vi "Strain Gauge Motion [FPGA Main].vi"() -> ()   [LabVIEW 2017]
doc: "Use this VI to control the cRIO Demo Kit motor and motor drive with a simple set of commands. You can operate the drive in 2 different modes. By default, you can input a velocity setpoint withing +20 or -20 rotations per second and the motor will move to that velocity, limited by the maximum acceleration input. Alternatively, you can turn on the heater mode. This will use the motor like a heater coil within the demo kit by setting the velocity to zero, but enabling full holding current through the drive. You can use the thermocouple in the demo kit to read the temperature of the motor windings. Turn the heating coil on and off by enabling and disabling the drive.\n\nUSING THIS VI: You can run this VI as the top level VI for an easy motion or heater component. Or you can modify this VI to run as a component of a main FPGA application. To do this, replace the front panel objects with target scoped registers, UDVs, or global variables."
uses:
  <vilib>/Platform/TimedLoop/XDataNode/timing_clust.ctl
  <vilib>/Platform/TimedLoop/XDataNode/nitl_modes.ctl
  <vilib>/Platform/TimedLoop/XDataNode/wakeup.ctl
  <vilib>/Motion/MotorControl/_s/nism.encoder.incremental.config.ctl
  <vilib>/Motion/MotorControl/_s/nism.incremental.indexCriteria.ctl
  <vilib>/LabVIEW Targets/FPGA/cRIO/shared/nicrio_ModuleControls/nicrio_cRIO-9503_DriveStatus.ctl
  <vilib>/Motion/MotorControl/_s/nism.stepper.currentScheduler.config.ctl
  <vilib>/Motion/MotorControl/_s/nism.microstepping.rate.ctl
  <vilib>/Motion/MotorControl/_s/nism.pi.gains.sgl.ctl
  <vilib>/Motion/MotorControl/_s/nism.pi.c.currentFeedback.sgl.ctl
  <vilib>/Motion/MotorControl/_s/nism.mdo.antiResonanceData.ctl
  <vilib>/Motion/MotorControl/_s/nism.stepper.currentScheduler.torqueSmoothingCoefficients.ctl
  <vilib>/Motion/MotorControl/_s/nism.pwm.outputs.4phase.ctl
  <vilib>/rvi/Emulation/niFpgaGetClockAttributes.vi
  <vilib>/rvi/Emulation/niFpgaSctlEmulationGetInTimedLoop.vi
  <vilib>/rvi/Emulation/niFpgaEmulationReportErrorSimple.vi
  <vilib>/rvi/eio/common/nirviEmuTemplateMethod_errors.vi
  <vilib>/rvi/Emulation/niFpgaCriticalErrorInLSC.vi
  <vilib>/rvi/DataTransferAndStorage/Container/Common/niFpgaContainerGetUniqueNameForEmu.vi
  <vilib>/rvi/DataTransferAndStorage/Container/Common/niFpgaContainerSetEmuInfo.vi
  <vilib>/rvi/eio/common/nirviEmuReportErrorAndStop.vi
  <vilib>/rvi/Emulation/niFpgaProcessEmulError.vi
  <vilib>/rvi/Emulation/niFpgaEmulationIsFPGAContextNoSignature.vi
  <vilib>/rvi/Memory/Memory_Emulation/niFpgaMemoryEmulationCacheClearOnFirstRun.vi
  <vilib>/rvi/Memory/Memory_Emulation/nirvimemoryEmulationManagerCache_MakeExclusive.vi
  <vilib>/rvi/Memory/Memory_Emulation/niFpgaMemoryEmulationValidateCache.vi
  <vilib>/rvi/Memory/Memory_Emulation/nirvimemoryEmulationManagerCache_InsertValue.vi
  <vilib>/Utility/error.llb/Clear Errors.vi
  <vilib>/rvi/Memory/Memory_Emulation/nirvimemoryEmulationManagerCache_ReleaseExclusive.vi
  <vilib>/rvi/Memory/Memory_Emulation/nirvimemoryEmulationManagerCache_GetValue.vi
  <vilib>/rvi/Memory/Memory_Emulation/nirvimemoryEmulationManagerCache_SetValue.vi
  <vilib>/Motion/MotorControl/_s/nism.incremental.p.2.vi
  <vilib>/rvi/occurrence/nirviWaitOnOccurrenceBase.vi
  <vilib>/Motion/MotorControl/_s/nism.rateLimiter.v.fxp.vi
  <vilib>/Motion/MotorControl/_s/nism.stepResolver.fxp.64.32.vi
  <vilib>/Motion/MotorControl/_s/nism.stepper.currentScheduler.advanced.single.vi
  <vilib>/Motion/MotorControl/_s/nism.pi.c.sgl.2phase.2.noAW.vi
  <vilib>/Motion/MotorControl/_s/nism.antiResonance.single.vi
  <vilib>/Motion/MotorControl/_s/nism.9503VoltageTransform.fxp.vi
  <vilib>/eio/EIONode/EIONode.xnode
  <vilib>/rvi/LocalResourceManager/LocalResourceManager.xnode
  <vilib>/rvi/DataTransferAndStorage/Container/XNode/niFpgaContainer.xnode
  <vilib>/rvi/DataTransferAndStorage/Register/Emulation/niFpgaRegisterEmulation.vi
  <vilib>/eio/EIOMethodNode/EIOMethodNode.xnode
  <vilib>/platform/TimedLoop/XDataNode/XDataNode.xnode
  <vilib>/Motion/MotorControl/NI_SoftMotion_MotorControlIP.lvlib
  <vilib>/Platform/TimedLoop/XDataNode/XDNodeRunTimeDep.lvlib
panel:
  out "Strain Gauge":sgl
  in  "Heater Mode":bool
  in  "Velocity Setpoint (rev/sec)":sgl caption="velocity setpoint"
  in  "Maximum Acceleration":T1(ring)=enum."High"
  out "Control Loop Timer":u32
  out "Anti-Resonance Enabled?":bool
  out "Pulse Per Revolution":bool
  out "Velocity (rev/sec)":fxp<+/-,32,16> caption="xi" format="%.41g"
  in  "Clear Faults":bool
  in  "Enable Drive":bool
  out "Module Fault Code":u16
  out "Module Fault?":bool
  # "Velocity is limited to +10 or -10 revolutions per second. Positive velocity setpoints equate to counter clockwise rotation.\n\nMax acceleration choices limit the rate of acceleration when changing velocity setpoints.\n\nHeater Mode will stop the motor and always keep full current through the motor windings, generating more heat.\n\nVelocity is the measured encoder velocity and works without the drive enabled. Pulse Per Revolution is the Z encoder pulse and occors exactly once for each revolution."
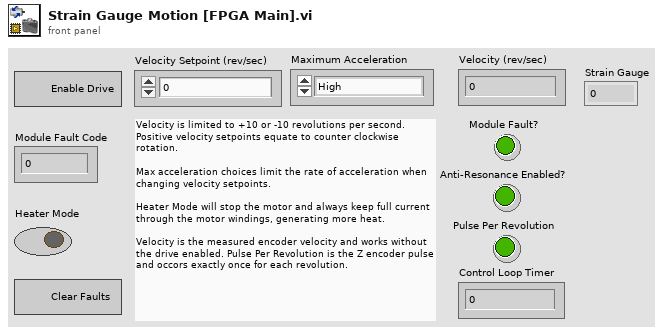
[diagram p1: front panel]
types:
  T1 = enum8{"Extremely Low", "Very Low", "Low", "Medium", "High", "Highest"}
  T2 = typedef "nicrio_cRIO-9503_DriveStatus.ctl" = enum8{"Drive Disabled (Disabled by fault)", "Drive Disabled (Disabled by software)", "Drive Enabled"}
  T3 = typedef "NI_SoftMotion_MotorControlIP.lvlib/nism.pwm.outputs.4phase.ctl" = cluster{"a+":fxp<+/-,16,1>, "a-":fxp<+/-,16,1>, "b+":fxp<+/-,16,1>, "b-":fxp<+/-,16,1>}
  T4 = typedef "XDNodeRunTimeDep.lvlib/timing_clust.ctl" = cluster{"Expected End [f-1]":u64, "Actual End [f-1]":u64, "Finished Late? [f-1]":bool, "Expected End [i-1]":u64, "Actual End [i-1]":u64, "Finished Late? [i-1]":bool, "Expected Start [i]":u64, "Actual Start [i]":u64, "Expected Start [f]":u64, "Actual Start [f]":u64, "Source Name":string, "Structure Name":string, "Period":i64, "Deadline":i64, "Offset":i64, "Start":i64, "Priority":i32, "Timeout":i32, "Mode":T5, "Wakeup Reason":T6, "Error":errorcluster, "Source Type":string, "Secondary Source Type":string, "Global End Time":u64, "Global Start Time":u64, "Frame Duration":u64, "Iteration Duration":u64, "Assigned CPU":i32, "I/O Scan Engine Mode":u32}
  T5 = typedef "XDNodeRunTimeDep.lvlib/nitl_modes.ctl" = enum32{"No Change", "Process missed periods, maintain original phase", "Discard missed periods, maintain original phase", "Process missed periods, ignore original phase", "Discard missed periods, ignore original phase"}
  T6 = typedef "XDNodeRunTimeDep.lvlib/wakeup.ctl" = enum32{"Normal", "Aborted", "Asynchronous wakeup", "Timing source error", "Timed loop error", "Timeout"}
  T7 = typedef "NI_SoftMotion_MotorControlIP.lvlib/nism.encoder.incremental.config.ctl" = cluster{"line a active high?":bool, "line b active high?":bool, "index active high?":bool}
  T8 = typedef "NI_SoftMotion_MotorControlIP.lvlib/nism.incremental.indexCriteria.ctl" = cluster{"a":bool, "b":bool, "z":bool}
  T9 = typedef "NI_SoftMotion_MotorControlIP.lvlib/nism.stepper.currentScheduler.torqueSmoothingCoefficients.ctl" = cluster{"current scheduler : torque smoothing : torque smoothing gain":sgl, "torque smoothing phase":fxp<+/-,16,1>}
  T10 = typedef "NI_SoftMotion_MotorControlIP.lvlib/nism.mdo.antiResonanceData.ctl" = cluster{"coefficient 0":sgl, "coefficient 1":sgl, "coefficient 2":sgl, "coefficient 3":sgl, "coefficient 4":sgl, "coefficient 5":sgl}
  T11 = typedef "NI_SoftMotion_MotorControlIP.lvlib/nism.pi.c.currentFeedback.sgl.ctl" = cluster{"phase a":sgl, "phase b":sgl}
  T12 = typedef "NI_SoftMotion_MotorControlIP.lvlib/nism.pi.gains.sgl.ctl" = cluster{"kp":sgl, "ki":sgl}
  T13 = typedef "NI_SoftMotion_MotorControlIP.lvlib/nism.microstepping.rate.ctl" = enum8{"1 (Full Step)", "2 (Half Step)", "4", "8", "16", "32", "64", "128", "256"}
  T14 = typedef "NI_SoftMotion_MotorControlIP.lvlib/nism.stepper.currentScheduler.config.ctl" = cluster{"rated phase current":sgl, "phase current offset(a)":sgl, "phase current offset(b)":sgl, "reduced current":sgl, "curr. reduction del.":u16}
  T15 = typedef "NI_SoftMotion_MotorControlIP.lvlib/nism.pi.c.currentSetpoint.sgl.ctl" = cluster{"phase a":sgl, "phase b":sgl}
  T16 = typedef "NI_SoftMotion_MotorControlIP.lvlib/nism.pi.c.voltage.sgl.ctl" = cluster{"phase a":sgl, "phase b":sgl}
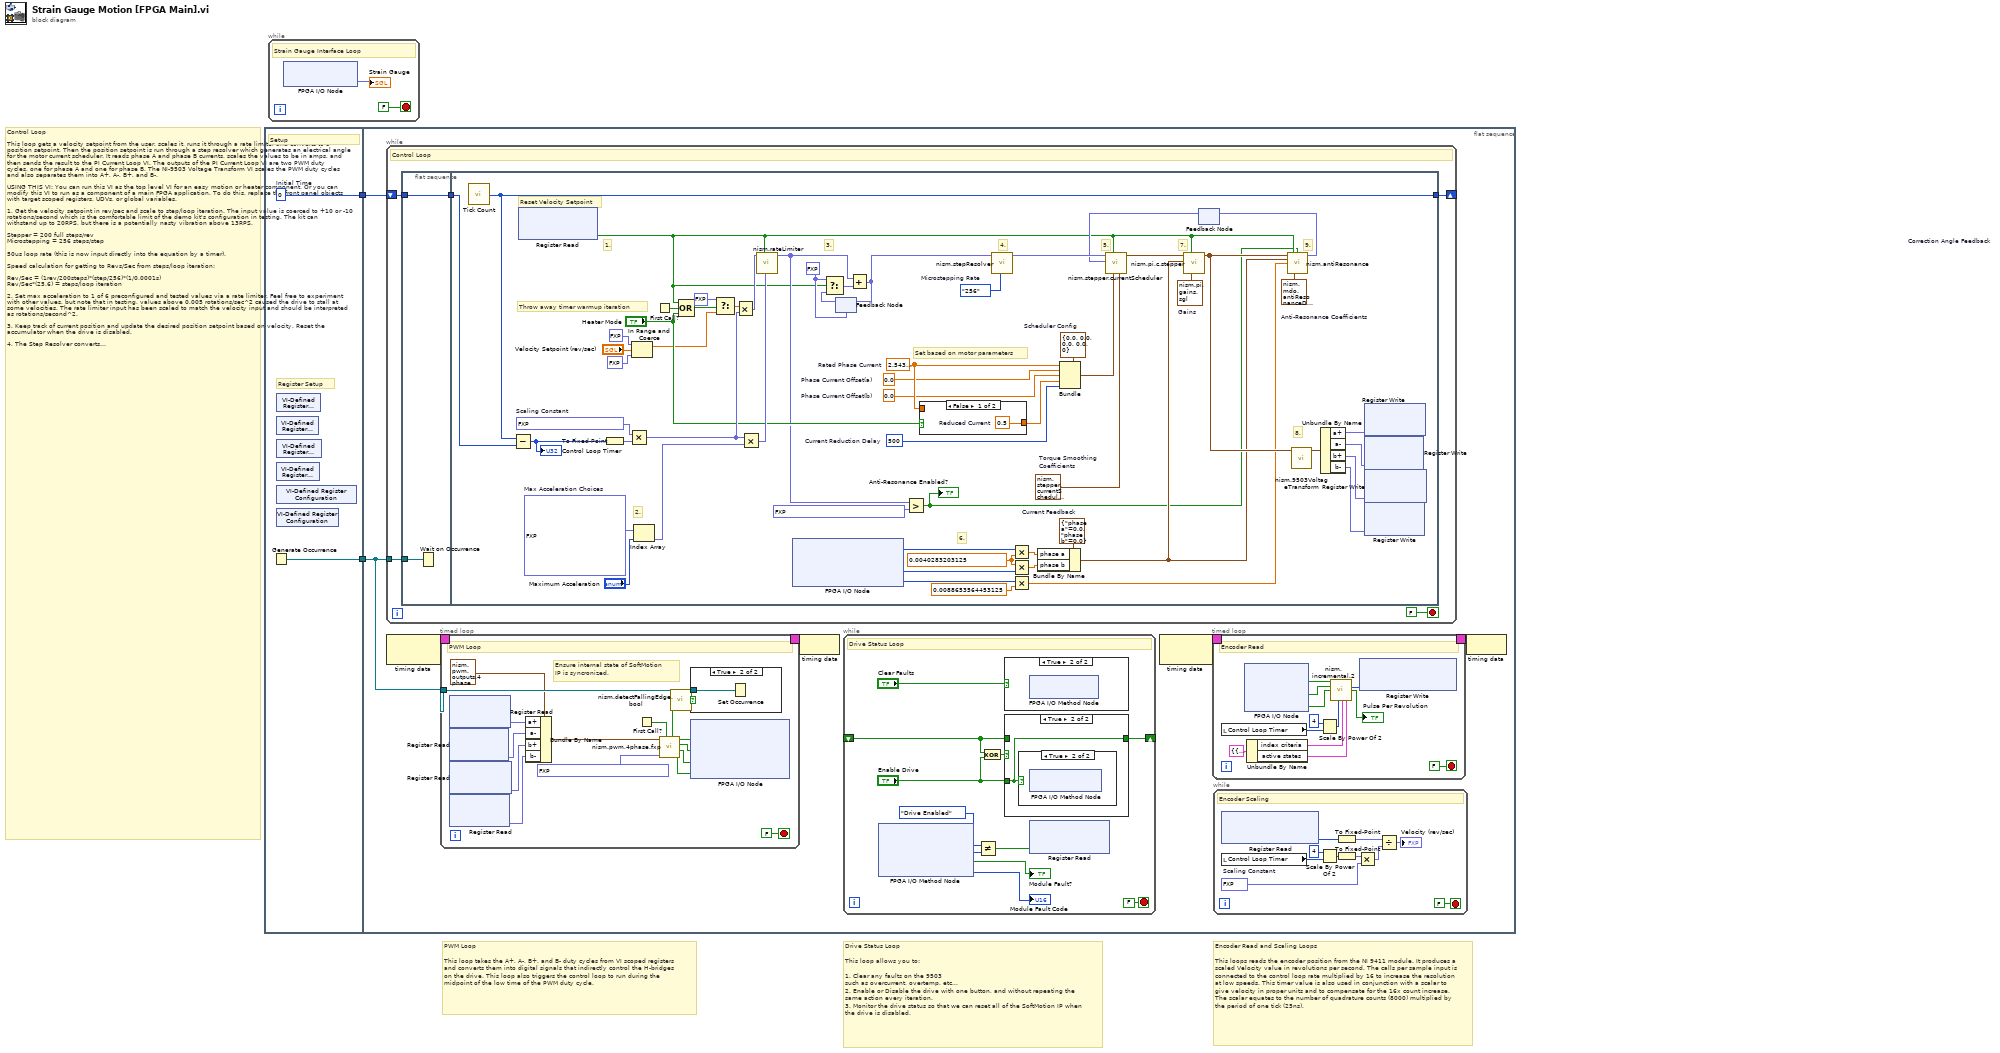
[diagram p0: block diagram]
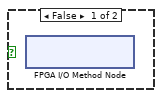
[diagram p4: hidden frame]
diagram:
  # "Encoder Read and Scaling Loops\n\nThis loops reads the encoder position from the NI 9411 module. It produces a scaled Velocity value in revolutions per second. The calls per sample input is connected to the control loop rate multiplied by 16 to increase the resolution at low speeds. This timer value is also used in conjunction with a scalar to give velocity in proper units and to compensate for the 16x count increase. The scalar equates to the number of quadrature counts (8000) multiplied by the period of one tick (25ns)."
  # "Drive Status Loop\n\nThis loop allows you to:\n \n1. Clear any faults on the 9503\nsuch as overcurrent, overtemp, etc...\n2. Enable or Disable the drive with one button, and without repeating the same action every iteration.\n3. Monitor the drive status so that we can reset all of the SoftMotion IP when the drive is disabled."
  # "PWM Loop\n\nThis loop takes the A+, A-, B+, and B- duty cycles from VI scoped registers and converts them into digital signals that indirectly control the H-bridges on the drive. This loop also triggers the control loop to run during the midpoint of the low time of the PWM duty cycle."
  # "Control Loop\n\nThis loop gets a velocity setpoint from the user, scales it, runs it through a rate limiter and converts to a position setpoint. Then the position setpoint is run through a step resolver which generates an electrical angle for the motor current scheduler. It reads phase A and phase B currents, scales the values to be in amps, and then sends the result to the PI Current Loop VI. The outputs of the PI Current Loop VI are two PWM duty cycles, one for phase A and one for phase B. The NI-9503 Voltage Transform VI scales the PWM duty cycles and also separates them into A+, A-, B+, and B-. \n\nUSING THIS VI: You can run this VI as the top level VI for an easy motion or heater component. Or you can modify this VI to run as a component of a main FPGA application. To do this, replace the front panel objects with target scoped registers, UDVs, or global variables.\n\n1. Get the velocity setpoint in rev/sec and scale to step/loop iteration. The input value is coerced to +10 or -10 rotations/second which is the comfortable limit of the demo kit's configuration in testing. The kit can withstand up to 20RPS, but there is a potentially nasty vibration above 13RPS.\n\nStepper = 200 full steps/rev\nMicrostepping = 256 steps/step\n\n50us loop rate (this is now input directly into the equation by a timer).\n\nSpeed calculation for getting to Revs/Sec from steps/loop iteration:\n\nRev/Sec = (1rev/200steps)*(step/256)*(1/0.0001s)\nRev/Sec*(25.6) = steps/loop iteration\n\n2. Set max acceleration to 1 of 6 preconfigured and tested values via a rate limiter. Feel free to experiment with other values, but note that in testing, values above 0.005 rotations/sec^2 caused the drive to stall at some velocities. The rate limiter input has been scaled to match the velocity input and should be interpreted as rotations/second^2. \n\n3. Keep track of current position and update the desired position setpoint based on velocity. Reset the accumulator when the drive is disabled.\n\n4. The Step Resolver converts a position setpoint to an electrical angle between -1 and 1 pi radians.\n\n5. The Motor Current Scheduler converts the electrical angle into phase A and phase B current setpoints. This is also where the rated phase current for the motor and the current reduction settings are implemented. Usually the motor current is reduced by a user-defined amount after a user-defined time period to save power and reduce temperature.  However, to use the motor as a heater for demo purposes with the attached thermocouple, there is an option to keep full current through the motor windings, generating heat. This is called \"heater mode.\" \n\n6. Read the phase A and phase B currents and scale them to be in amps. The current read is triggered by the PWM loop.\n\n7. Run the PI Current Loop to get two PWM duty cycles, one for phase A and one for phase B.  Current control loop gains are calculated based on motor parameters.\n \n8. Scale the PWM duty cycles and split them into four different duty cycles: A+, A-, B+, and B-. Send those duty cycles to the PWM Loop via registers.\n\n9. Applies an anti-resonance algorithm to reduce resonance of the stepper motor allowing for increased speed and performance."
  n1 = flat-sequence {
    tunnel: [w4] -> w2
    tunnel: [w3] -> w1
    tunnel: w2 -> [w6]
    tunnel: w1 -> [w5]
    frame #0 {
      w3 = u32 0  # Initial Time
      # "Setup"
      # "Register Setup"
      # "Setup"
      n2 = Generate Occurrence() -> (w4:refnum<k4>)
      n3 = xnode ("VI-Defined Register Configuration")() -> ()  [unwired: 1 out]
      n4 = xnode ("VI-Defined Register Configuration")() -> ()  [unwired: 1 out]
      n5 = xnode ("VI-Defined Register Configuration")() -> ()  [unwired: 1 out]
      n6 = xnode ("VI-Defined Register Configuration")() -> ()  [unwired: 1 out]
      n7 = xnode ("VI-Defined Register Configuration")() -> ()  [unwired: 1 out]
      n8 = xnode ("VI-Defined Register Configuration")() -> ()  [unwired: 1 out]
    }
    frame #1 {
      n9 = while "Control Loop" {
        tunnel: w6 -> [w75]
        shift-right: [w71] -> _
        shift-left: w5 -> [w73]
        stop <- FALSE stop-if-true
        # "Control Loop"
        n10 = flat-sequence {
          tunnel: w75 -> [w77]
          tunnel: [w76] -> w72
          tunnel: w73 -> [w76]
          tunnel: [w136] -> w71
          tunnel: w72 -> [w124]
          frame #0 {
            n11 = Wait on Occurrence(2:w77) -> ()  [unwired: 2 in, 1 out]
          }
          frame #1 {
            w81 = T9 {"current scheduler : torque smoothing : torque smoothing gain"=0.054, "torque smoothing phase"=-0.13800048828125}  # Torque Smoothing Coefficients
            w84 = T10 {"coefficient 0"=0.5555556, "coefficient 1"=0.98511136, "coefficient 2"=0.007444307, "coefficient 3"=1.0, "coefficient 4"=0.9812323, "coefficient 5"=0.009383864}  # Anti-Resonance Coefficients
            w93 = T11 {"phase a"=0.0, "phase b"=0.0}  # Current Feedback
            w94 = T12 {"kp"=1.57, "ki"=0.0235}  # Gains
            w102 = sgl 0.0040283203 ("y")
            w110 = fxp<+/-,32,16>[] [1.52587890625e-05, 4.57763671875e-05, 0.0001068115234375, 0.0005035400390625, 0.001007080078125, 0.0050048828125]  # Max Acceleration Choices
            w116 = fxp<+/-,64,32> 0.0 ("t")
            w123 = fxp<+,16,-9> 0.0012800097465515137  # Scaling Constant
            w91 = nism.microstepping.rate."256"  # Microstepping Rate
            w135 = T14 {"rated phase current"=0.0, "phase current offset(a)"=0.0, "phase current offset(b)"=0.0, "reduced current"=0.0, "curr. reduction del."=0}  # Scheduler Config
            w132 = u16 500  # Current Reduction Delay
            w131 = sgl 0.0  # Phase Current Offset(b)
            w130 = sgl 0.0  # Phase Current Offset(a)
            w134 = sgl 2.544  # Rated Phase Current
            # "9."
            # "Throw away timer warmup iteration"
            # "Reset Velocity Setpoint"
            # "3."
            # "2."
            # "1."
            # "Set based on motor parameters"
            # "5."
            # "4."
            # "6."
            # "8."
            # "7."
            n12 = call "Tick Count"() -> ("Tick Count(Ticks)"=w136:u32)
            n13 = Subtract(x=w136, y=w124) -> (x-y=w96:u32)
            "Control Loop Timer" <- w96
            n14 = xnode ("Register Read")() -> ("Data"=w79:bool)  [unwired: 1 in, 1 out]
            n15 = To Fixed-Point(number=w96) -> (fixed-point=w97:fxp<+,16,16>)  [unwired: 1 in]
            n16 = Multiply(x=w123, y=w97) -> (x*y=w122:fxp<+,32,16>)
            n17 = In Range and Coerce(upper limit=fxp<+/-,32,16> 10.0, x="Velocity Setpoint (rev/sec)", lower limit=fxp<+/-,32,16> -10.0) -> (coerced(x)=w113:sgl)  [unwired: 1 out]
            n18 = Index Array(array=w110, index="Maximum Acceleration") -> (element=w108:fxp<+/-,32,16>)
            n19 = First Call?() -> (First Call?: T/F=w120:bool)
            n20 = Compound Arithmetic op=OR(w79, w120, "Heater Mode") -> (w119:bool)
            n21 = Select(t=fxp<+/-,32,16> 0.0, s=w119, f=w113) -> (s? t:f=w126:sgl)
            n22 = Multiply(x=w126, y=w122) -> (x*y=w128:fxp<+/-,64,32>)
            n23 = Multiply(x=w122, y=w108) -> (x*y=w127:fxp<+/-,64,32>)
            n24 = call-poly <vilib>:"nism.rateLimiter.vi"("max acceleration"=w127, "reset"=w79, "velocity setpoint"=w128) -> ("limited velocity"=w80:fxp<+/-,64,32>)  [unwired: 8 in]
            n25 = xnode "FPGA I/O Node"() -> ("Mod1/Phase A Current"=w99:i16, "Mod1/Phase B Current"=w98:i16, "Mod1/Vsup Voltage"=w88:u16)  [unwired: 3 in, 3 out]
            n26 = feedback #1(w116) -> (w117:fxp<+/-,64,32>)
            n27 = Select(t=w116, s=w79, f=w117) -> (s? t:f=w118:fxp<+/-,64,32>)
            n28 = Add(x=w80, y=w118) -> (x+y=w115:fxp<+/-,64,32>)
            n29 = feedback-in #1(w115) -> ()
            n30 = Greater?(x=w80, y=fxp<+/-,64,32> 5.120000000111759) -> (0:w78:bool)
            "Anti-Resonance Enabled?" <- w78
            n31 = case shown="False" "Heater Mode" {
              tunnel: [w137 w138] -> w133
              tunnel: w134 -> [_ w138]
              frame False {
                w137 = sgl 0.5  # Reduced Current
              }
              frame True {
              }
            }
            n32 = call-poly <vilib>:"nism.stepResolver.vi"("microstepping rate"=w91, "position setpoint"=w115) -> ("electrical angle"=w129:fxp<+/-,16,1>)  [unwired: 9 in]
            n33 = Multiply(x=w99, y=w102) -> (x*y=w101:sgl)
            n34 = Multiply(x=w102, y=w98) -> (x*y=w100:sgl)
            n35 = Multiply(x=w88, y=sgl 0.008865356 ("orig 9503")) -> (x*y=w86:sgl)
            n36 = Bundle By Name(cluster=w93, "phase a"=w101, "phase b"=w100) -> (w89:T11)
            n37 = Bundle(cluster=w135, "rated phase current"=w134, "phase current offset(a)"=w130, "phase current offset(b)"=w131, "reduced current"=w133, "curr. reduction del."=w132) -> (w92:T14)
            n38 = feedback #2 "Correction Angle Feedback"() -> (w82:fxp<+/-,16,1>)  [unwired: 1 in]
            n39 = call-poly <vilib>:"nism.stepper.currentScheduler.vi"("torque smoothing coefficients"=w81, "current scheduler config"=w92, "reset"=w79, "correction angle"=w82, "electrical angle"=w129) -> ("current setpoint"=w95:T15)  [unwired: 6 in]
            n40 = call-poly <vilib>:"nism.pi.c.stepper.vi"("gains"=w94, "reset"=w79, "current feedback"=w89, "current setpoint"=w95) -> ("voltage output"=w90:T16)  [unwired: 6 in, 1 out]
            n41 = call-poly <vilib>:"nism.antiResonance.vi"("voltage output"=w90, "reset"=w79, "enable"=w78, "current feedback"=w89, "bus voltage"=w86, "anti-resonance coefficients"=w84) -> ("correction angle"=w83:fxp<+/-,16,1>)  [unwired: 9 in]
            n42 = feedback-in #2(w83) -> ()
            n43 = call-poly <vilib>:"nism.9503VoltageTransform.vi"("voltage output"=w90) -> ("duty cycles"=w107:T3)  [unwired: 10 in]
            n44 = Unbundle By Name(w107) -> ("a+"=w106:fxp<+/-,16,1>, "a-"=w105:fxp<+/-,16,1>, "b+"=w104:fxp<+/-,16,1>, "b-"=w103:fxp<+/-,16,1>)
            n45 = xnode ("Register Write")("Data"=w106) -> ()  [unwired: 1 in, 1 out]
            n46 = xnode ("Register Write")("Data"=w105) -> ()  [unwired: 1 in, 1 out]
            n47 = xnode ("Register Write")("Data"=w104) -> ()  [unwired: 1 in, 1 out]
            n48 = xnode ("Register Write")("Data"=w103) -> ()  [unwired: 1 in, 1 out]
          }
        }
      }
      n49 = node-c288() -> (w8:T4)  [unwired: 1 in]
      n50 = timed-loop "PWM Loop" {
        timing: w8 -> [_]
        timing-out: [_] -> w7
        tunnel: w6 -> [w32]
        stop <- FALSE stop-if-true
        # "Ensure internal state of SoftMotion\nIP is syncronized."
        # "PWM Loop"
        n51 = xnode ("Register Read")() -> ("Data"=w29:fxp<+/-,16,1>)  [unwired: 1 in, 1 out]
        n52 = xnode ("Register Read")() -> ("Data"=w28:fxp<+/-,16,1>)  [unwired: 1 in, 1 out]
        n53 = xnode ("Register Read")() -> ("Data"=w27:fxp<+/-,16,1>)  [unwired: 1 in, 1 out]
        n54 = xnode ("Register Read")() -> ("Data"=w26:fxp<+/-,16,1>)  [unwired: 1 in, 1 out]
        n55 = Bundle By Name(cluster=T3 {"a+"=0.0, "a-"=0.0, "b+"=0.0, "b-"=0.0} ("duty cycles"), "a+"=w29, "a-"=w28, "b+"=w27, "b-"=w26) -> (w30:T3)
        n56 = First Call?() -> (First Call?: T/F=w24:bool)
        n57 = call <vilib>:"nism.pwm.4phase.fxp.vi"("reset"=w24, "frequency"=fxp<+,32,0> 0.0005000000819563866, "duty cycles"=w30) -> ("phase b-"=w35:bool, "phase b+"=w36:bool, "phase a-"=w37:bool, "phase a+"=w38:bool, "trigger"=w34:bool)  [unwired: 4 in]
        n58 = call <vilib>:"nism.detectFallingEdge.bool.vi"("x"=w34) -> ("y"=w33:bool)
        n59 = case shown="True" w33 {
          tunnel: w32 -> [_ w40]
          frame False {
          }
          frame True {
            n60 = Set Occurrence(w40) -> ()
          }
        }
        n61 = xnode "FPGA I/O Node"("Mod1/Phase A Pos"=w38, "Mod1/Phase A Neg"=w37, "Mod1/Phase B Pos"=w36, "Mod1/Phase B Neg"=w35) -> ()  [unwired: 4 in, 4 out]
      }
      n62 = node-c288(w7) -> ()
      n63 = while "Drive Status Loop" {
        shift-right: [w19] -> _
        shift-left: _ -> [w18]
        stop <- FALSE stop-if-true
        # "Drive Status Loop"
        n64 = xnode "FPGA I/O Method Node"() -> ("Drive Status"=w15:T2, "Module Fault?"=→"Module Fault?":bool, "Module Fault Code"=→"Module Fault Code":u16)  [unwired: 1 in, 1 out]
        n65 = Not Equal?(x=nicrio_cRIO-9503_DriveStatus."Drive Enabled" ("y"), y=w15) -> (x != y?=w13:bool)
        n66 = Exclusive Or(1:"Enable Drive", 2:w18) -> (0:w20:bool)
        n67 = case shown="True" "Clear Faults" {
          frame False {
          }
          frame True {
            n68 = xnode "FPGA I/O Method Node"() -> ()  [unwired: 1 in, 1 out]
          }
        }
        n69 = case shown="True" w20 {
          tunnel: "Enable Drive" -> [_ w23]
          tunnel: [w22 w23] -> w19
          tunnel: w18 -> [w22 _]
          frame False {
          }
          frame True {
            n70 = case shown="True" w23 {
              frame False {
                n71 = xnode "FPGA I/O Method Node"() -> ()  [unwired: 1 in, 1 out]
              }
              frame True {
                n72 = xnode "FPGA I/O Method Node"() -> ()  [unwired: 1 in, 1 out]
              }
            }
          }
        }
        n73 = xnode ("Register Read")("Data"=w13) -> ()  [unwired: 1 in, 1 out]
      }
      n74 = node-c288() -> (w10:T4)  [unwired: 1 in]
      n75 = timed-loop "Encoder Read" {
        timing: w10 -> [_]
        timing-out: [_] -> w9
        stop <- FALSE stop-if-true
        # "Encoder Read"
        n76 = local read "Control Loop Timer"() -> (w57:u32)
        n77 = xnode "FPGA I/O Node"() -> ("EncoderA"=w61:bool, "EncoderB"=w60:bool, "EncoderZ"=w59:bool)  [unwired: 3 in, 3 out]
        n78 = Unbundle By Name(cluster{"active states":T7, "index criteria":T8} {"active states"={"line a active high?"=TRUE, "line b active high?"=TRUE, "index active high?"=TRUE}, "index criteria"={"a"=FALSE, "b"=FALSE, "z"=TRUE}} ("Encoder Config")) -> ("index criteria"=w65:T8, "active states"=w64:T7)
        n79 = Scale By Power Of 2(n=i16 4, x=w57) -> (x*2^n=w56:u32)
        n80 = call-poly <vilib>:"nism.incremental.2.vi"("a phase"=w61, "b phase"=w60, "z phase"=w59, "calls per sample"=w56, "index criteria"=w65, "active states"=w64) -> ("velocity"=w58:i16, "index"=→"Pulse Per Revolution":bool)  [unwired: 6 in, 2 out]
        n81 = xnode ("Register Write")("Data"=w58) -> ()  [unwired: 1 in, 1 out]
      }
      n82 = while "Encoder Scaling" {
        stop <- FALSE stop-if-true
        w52 = fxp<+,8,-12> 0.0002002716064453125  # Scaling Constant
        # "Encoder Scaling"
        n83 = local read "Control Loop Timer"() -> (w48:u32)
        n84 = xnode ("Register Read")() -> ("Data"=w50:i16)  [unwired: 1 in, 1 out]
        n85 = Scale By Power Of 2(n=i16 4, x=w48) -> (x*2^n=w46:u32)
        n86 = To Fixed-Point(number=w50) -> (fixed-point=w49:fxp<+/-,32,16>)  [unwired: 1 in]
        n87 = To Fixed-Point(number=w46) -> (fixed-point=w45:fxp<+,16,16>)  [unwired: 1 in]
        n88 = Multiply(x=w45, y=w52) -> (x*y=w54:fxp<+/-,32,16>)
        n89 = Divide(x=w49, y=w54) -> (x/y=→"Velocity (rev/sec)":fxp<+/-,32,16>)
      }
      n90 = node-c288(w9) -> ()
    }
  }
  n91 = while {
    stop <- FALSE stop-if-true
    # "Strain Gauge Interface Loop"
    n92 = xnode "FPGA I/O Node"() -> ("Strain Gauge"=→"Strain Gauge":fxp<+/-,32,7>)  [unwired: 1 in, 1 out]
  }
